vi "Add Library To Project.vi"(8 "error in":errorcluster, 10 "library path":path, 11 "configuration":T1) -> (0 "error out":errorcluster, 3 "project ref out":refnum<vi>)   [LabVIEW 2021, in "InstrumentStudio Plug-In Editor.lvlib"]
uses:
  InstrumentStudio Plug-In Editor.lvlib
  Data Holder.ctl
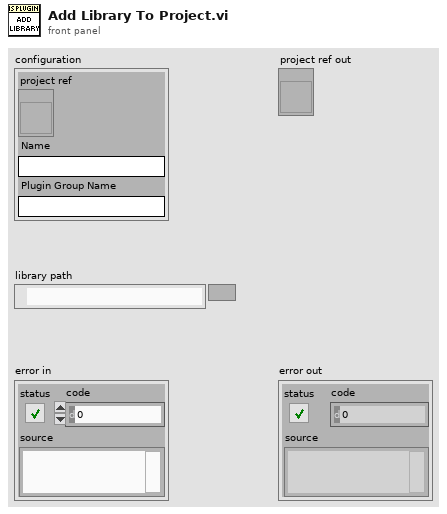
[diagram p1: front panel]
types:
  T1 = typedef "InstrumentStudio Plug-In Editor.lvlib/Data Holder.ctl" = cluster{"project ref":refnum<vi>, "Name":string, "Plugin Group Name":string}
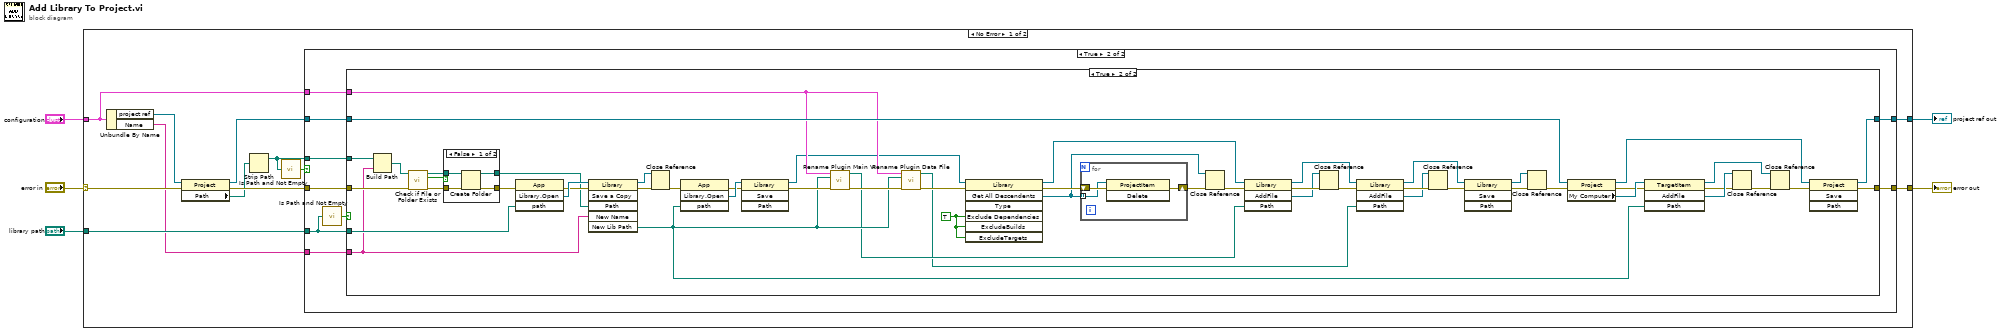
[diagram p0: block diagram]
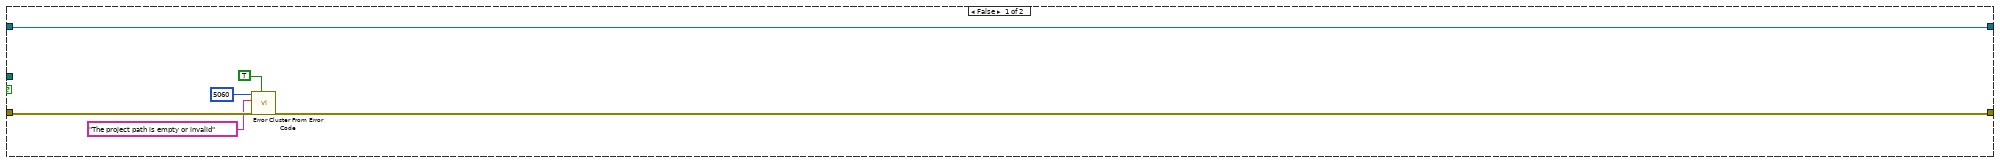
[diagram p2: hidden frame]
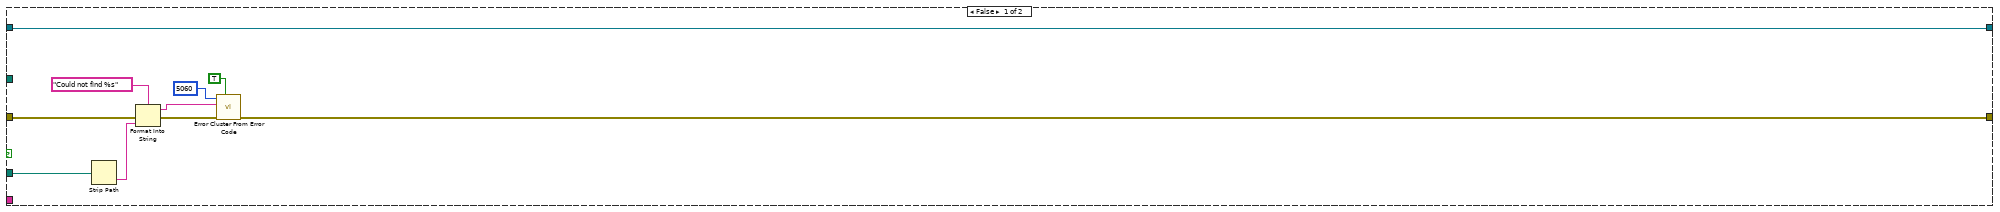
[diagram p3: hidden frame]
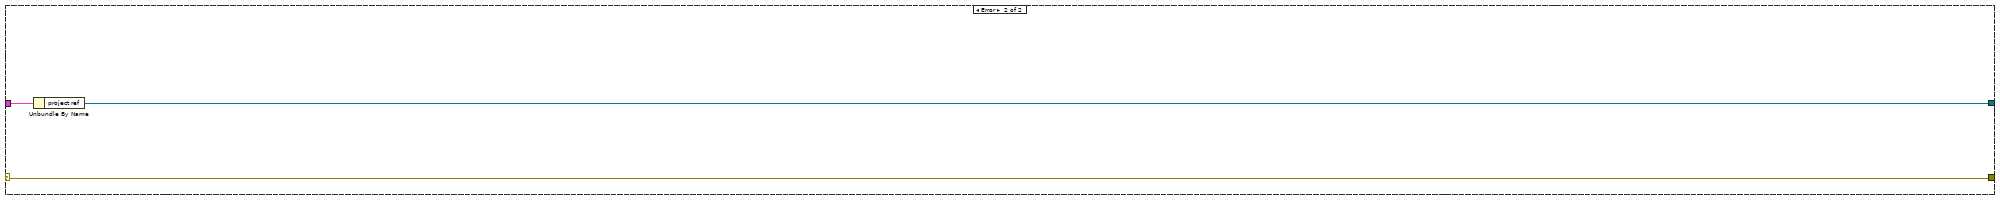
[diagram p5: hidden frame]
diagram:
  n1 = case shown="No Error" "error in" {
    selector: "error in" -> [w11 w106]
    tunnel: "library path" -> [w16 _]
    tunnel: [w15 w107] -> w5
    tunnel: "configuration" -> [w13 w105]
    tunnel: [w9 w106] -> w4
    frame No Error {
      n2 = Unbundle By Name(w13) -> ("project ref"=w14:refnum<vi>, "Name"=w8:string)
      n3 = property class="Project"(reference=w14, error in=w11) -> (reference out=w12:refnum<vi>, error out=w10:errorcluster, "Path"=w6:path)
      n4 = Strip Path(path=w6) -> (stripped path=w7:path)  [unwired: 1 out]
      n5 = call <vilib>:"Is Path and Not Empty.vi"("path"=w7) -> ("Is Path and Not Empty?"=w17:bool)  [unwired: 4 in]
      n6 = case shown="True" w17 {
        tunnel: w16 -> [_ w24]
        tunnel: w8 -> [_ w32]
        tunnel: w7 -> [_ w31]
        tunnel: [w23 w30] -> w15
        tunnel: w13 -> [_ w29]
        tunnel: w12 -> [w23 w28]
        tunnel: w10 -> [w22 w26]
        tunnel: [w18 w25] -> w9
        frame False {
          n7 = call <vilib>:"Error Cluster From Error Code.vi"("show call chain? (False)"=TRUE, "error in (no error)"=w22, "error message (\"\")"="The project path is empty or invalid" ("error message (\"\")"), "error code (0)"=5060) -> ("error out"=w18:errorcluster)  [unwired: 5 in]
        }
        frame True {
          n8 = call <vilib>:"Is Path and Not Empty.vi"("path"=w24) -> ("Is Path and Not Empty?"=w27:bool)  [unwired: 4 in]
          n9 = case shown="True" w27 {
            tunnel: w24 -> [w33 w69]
            tunnel: w32 -> [_ w68]
            tunnel: w31 -> [_ w95]
            tunnel: [w40 w93] -> w30
            tunnel: w29 -> [_ w65]
            tunnel: w28 -> [w40 w83]
            tunnel: w26 -> [w37 w92]
            tunnel: [w34 w79] -> w25
            frame False {
              n10 = Strip Path(path=w33) -> (name=w38:string)  [unwired: 1 out]
              n11 = Format Into String(format string="Could not find %s", error in=w37, w38) -> (resulting string=w41:string, error out=w42:errorcluster)  [unwired: 1 in]
              n12 = call <vilib>:"Error Cluster From Error Code.vi"("show call chain? (False)"=TRUE, "error in (no error)"=w42, "error message (\"\")"=w41, "error code (0)"=5060) -> ("error out"=w34:errorcluster)  [unwired: 5 in]
            }
            frame True {
              w47 = TRUE ("ExcludeDependencies")
              n13 = Build Path(base path=w95, name or relative path=w68) -> (appended path=w94:path)
              n14 = call <vilib>:"Check if File or Folder Exists.vi"("error in (no error)"=w92, "path"=w94) -> ("error out"=w91:errorcluster, "file or folder exists?"=w89:bool, "dup path"=w90:path)  [unwired: 7 in]
              n15 = case shown="False" w89 {
                tunnel: w91 -> [w102 w103]
                tunnel: w90 -> [w101 w104]
                tunnel: [w100 w104] -> w70
                tunnel: [w99 w103] -> w71
                frame False {
                  n16 = Create Folder(path (use dialog)=w101, error in=w102) -> (created path=w100:path, error out=w99:errorcluster)  [unwired: 1 in, 1 out]
                }
                frame True {
                }
              }
              n17 = invoke class="App" method="Library.Open"(error in=w71, "path"=w69) -> (error out=w75:errorcluster, "Open Library"=w78:refnum<vi>)  [unwired: 2 in, 2 out]
              n18 = invoke class="Library" method="Save a Copy"(reference=w78, error in=w75, "Path"=w70, "New Name"=w68) -> (reference out=w77:refnum<vi>, error out=w74:errorcluster, "New Lib Path"=w50:path)  [unwired: 2 in, 3 out]
              n19 = Close Reference(reference=w77, error in (no error)=w74) -> (error out=w73:errorcluster)
              n20 = invoke class="App" method="Library.Open"(error in=w73, "path"=w50) -> (error out=w72:errorcluster, "Open Library"=w76:refnum<vi>)  [unwired: 2 in, 2 out]
              n21 = invoke class="Library" method="Save"(reference=w76, error in=w72) -> (reference out=w62:refnum<vi>, error out=w67:errorcluster)  [unwired: 2 in, 2 out]
              n22 = call "Rename Plugin Main VI.vi"("configuration"=w65, "Plugin Library Path"=w50, "error in"=w67) -> ("Plugin Main VI Path"=w49:path, "error out"=w66:errorcluster)  [unwired: 11 in]
              n23 = call "Rename Plugin Data File.vi"("configuration"=w65, "Plugin Library Path"=w50, "error in"=w66) -> ("Plugin Data File Path"=w48:path, "error out"=w64:errorcluster)  [unwired: 11 in]
              n24 = invoke class="Library" method="Get All Descendents"(reference=w62, error in=w64, "Exclude Dependencies"=w47, "ExcludeBuilds"=w47, "ExcludeTargets"=w47) -> (reference out=w46:refnum<vi>, error out=w63:errorcluster, "All Descendents"=w59:refnum<vi>[])  [unwired: 2 in, 4 out]
              n25 = for {
                shift-right: [w97] -> w61
                shift-left: w63 -> [w98]
                tunnel: w59 -> [w96] mode=indexing
                n26 = invoke class="ProjectItem" method="Delete"(reference=w96, error in=w98) -> (error out=w97:errorcluster)  [unwired: 1 in, 2 out]
              }
              n27 = Close Reference(reference=w59, error in (no error)=w61) -> (error out=w60:errorcluster)
              n28 = invoke class="Library" method="AddFile"(reference=w46, error in=w60, "Path"=w49) -> (reference out=w43:refnum<vi>, error out=w58:errorcluster, "AddFile"=w44:refnum<vi>)  [unwired: 1 in, 1 out]
              n29 = Close Reference(reference=w44, error in (no error)=w58) -> (error out=w45:errorcluster)
              n30 = invoke class="Library" method="AddFile"(reference=w43, error in=w45, "Path"=w48) -> (reference out=w53:refnum<vi>, error out=w57:errorcluster, "AddFile"=w55:refnum<vi>)  [unwired: 1 in, 1 out]
              n31 = Close Reference(reference=w55, error in (no error)=w57) -> (error out=w56:errorcluster)
              n32 = invoke class="Library" method="Save"(reference=w53, error in=w56) -> (reference out=w51:refnum<vi>, error out=w54:errorcluster)  [unwired: 2 in, 2 out]
              n33 = Close Reference(reference=w51, error in (no error)=w54) -> (error out=w52:errorcluster)
              n34 = property class="Project"(reference=w83, error in=w52) -> (reference out=w80:refnum<vi>, error out=w86:errorcluster, "My Computer"=w88:refnum<vi>)
              n35 = invoke class="TargetItem" method="AddFile"(reference=w88, error in=w86, "Path"=w50) -> (reference out=w81:refnum<vi>, error out=w85:errorcluster, "AddFile"=w87:refnum<vi>)  [unwired: 1 in, 1 out]
              n36 = Close Reference(reference=w87, error in (no error)=w85) -> (error out=w84:errorcluster)
              n37 = Close Reference(reference=w81, error in (no error)=w84) -> (error out=w82:errorcluster)
              n38 = invoke class="Project" method="Save"(reference=w80, error in=w82) -> (reference out=w93:refnum<vi>, error out=w79:errorcluster)  [unwired: 2 in, 2 out]
            }
          }
        }
      }
    }
    frame Error {
      n39 = Unbundle By Name(w105) -> ("project ref"=w107:refnum<vi>)
    }
  }
  "error out" <- w4
  "project ref out" <- w5
